vi "Read Value (variant).vi"(8 "error in (no error)":errorcluster, 11 "Ring D Element in":refnum<class "String dropdown D Element.lvclass">) -> (0 "error out":errorcluster, 2 "Variant":variant, 3 "Ring D Element out":refnum<class "String dropdown D Element.lvclass">)   [LabVIEW 2018, in "D Datagrid Library.lvlib" / "String dropdown D Element.lvclass"]
uses:
  String dropdown D Element.lvclass
  String dropdown D Element.lvclass/String dropdown D Element.ctl
  Read value.vi
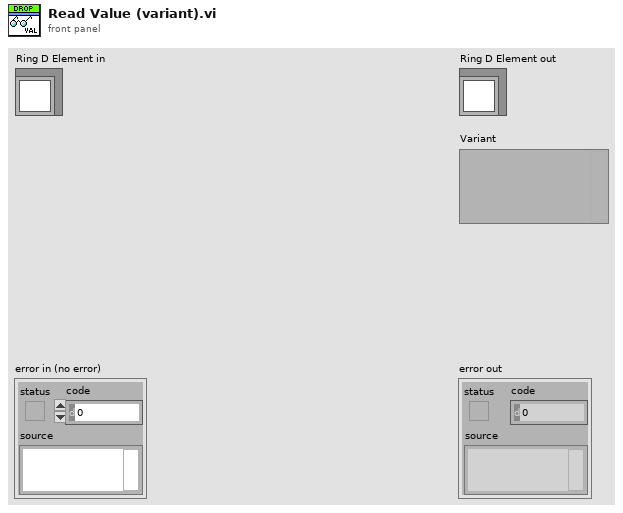
[diagram p1: front panel]
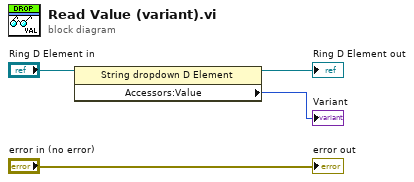
[diagram p0: block diagram]
diagram:
  n1 = property class="String dropdown D Element"(reference="Ring D Element in") -> (reference out=→"Ring D Element out":refnum<class "String dropdown D Element.lvclass">, "Accessors:Value"=→"Variant":i32)  [unwired: 1 in, 1 out]
  "error out" <- "error in (no error)"
